vi "Update Channel (implicit).vi"(8 "error in (no error)":errorcluster, 10 "Channel":refnum<class "Channel.lvclass">, 11 "SignalManager in":refnum<class "SignalManager.lvclass">) -> (0 "error out":errorcluster, 3 "SignalManager out":refnum<class "SignalManager.lvclass">)   [LabVIEW 2015, in "SignalManager.lvclass"]
uses:
  SignalManager.lvclass
  Channel/Channel.lvclass
  SignalManager.lvclass/SignalManager.ctl
  Channel/Channel.lvclass/Channel.ctl
  Channel/Read Name.vi
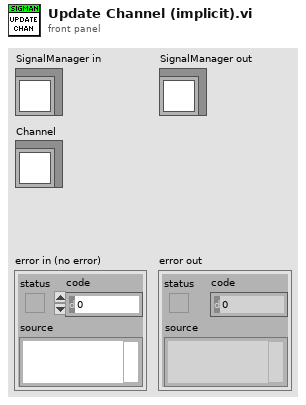
[diagram p1: front panel]
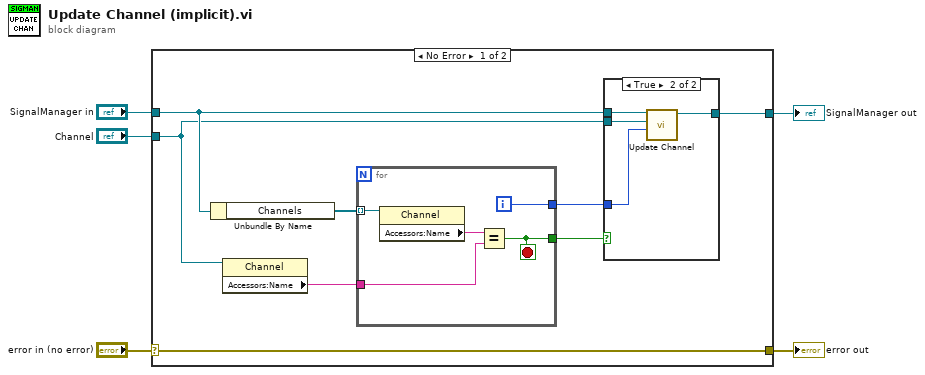
[diagram p0: block diagram]
diagram:
  n1 = case shown="No Error" "error in (no error)" {
    selector: "error in (no error)" -> [w13 w25]
    tunnel: [w13 w25] -> w4
    tunnel: [w6 w24] -> w2
    tunnel: "SignalManager in" -> [w10 w24]
    tunnel: "Channel" -> [w9 _]
    frame No Error {
      n2 = Unbundle By Name(w10) -> ("Channels"=w12:refnum<class "Channel.lvclass">[])
      n3 = property class="Channel"(reference=w9) -> ("Accessors:Name"=w11:string)  [unwired: 1 in, 2 out]
      n4 = for {
        tunnel: w12 -> [w23] mode=indexing
        tunnel: w11 -> [w21]
        tunnel: [w20] -> w8
        tunnel: [w19] -> w7
        i -> [w20]
        stop <- w19 stop-if-true
        n5 = property class="Channel"(reference=w23) -> ("Accessors:Name"=w22:string)  [unwired: 1 in, 2 out]
        n6 = Equal?(x=w22, y=w21) -> (x = y?=w19:bool)
      }
      n7 = case shown="True" w7 {
        tunnel: w10 -> [w14 w18]
        tunnel: w9 -> [_ w17]
        tunnel: w8 -> [_ w16]
        tunnel: [w14 w15] -> w6
        frame False {
        }
        frame True {
          n8 = call "Update Channel.vi"("Channel Index"=w16, "Channel"=w17, "SignalManager in"=w18) -> ("SignalManager out"=w15:refnum<class "SignalManager.lvclass">)  [unwired: 7 in, 1 out]
        }
      }
    }
    frame Error {
    }
  }
  "error out" <- w4
  "SignalManager out" <- w2
